vi "sv_Insert Swept THD Values.vi"(8 "scaled measurements in":T1 {"harmonic components [ratio]" format="%.2f"; "THD [ratio]" format="%.2f"; "FRF Measurements"."Im [response]" format="%.2f"; "FRF Measurements"."Re [response]" format="%.2f"; "FRF Measurements"."Im [stimulus]" format="%.2f"; "FRF Measurements"."Re [stimulus]" format="%.2f"; "RMS response" format="%.2f"; "RMS stimulus" format="%.2f"}, 10 "AI freq index":i32, 11 "measurements in":T2 {"scaled response magnitude" format="%.3f"; "Harm[]" format="%.2f"; "THD" format="%.2f"; "Im [response]" format="%.2f"; "Re [response]" format="%.2f"; "Im [stimulus]" format="%.2f"; "Re [stimulus]" format="%.2f"; "RMS response" format="%.2f"; "RMS stimulus" format="%.2f"}) -> (0 "dup new measurements":T1 {"harmonic components [ratio]" format="%.2f"; "THD [ratio]" format="%.2f"; "FRF Measurements"."Im [response]" format="%.2f"; "FRF Measurements"."Re [response]" format="%.2f"; "FRF Measurements"."Im [stimulus]" format="%.2f"; "FRF Measurements"."Re [stimulus]" format="%.2f"; "RMS response" format="%.2f"; "RMS stimulus" format="%.2f"}, 2 "dup AI freq index":i32, 3 "measurements out":T2 {"scaled response magnitude" format="%.3f"; "Harm[]" format="%.2f"; "THD" format="%.2f"; "Im [response]" format="%.2f"; "Re [response]" format="%.2f"; "Im [stimulus]" format="%.2f"; "Re [stimulus]" format="%.2f"; "RMS response" format="%.2f"; "RMS stimulus" format="%.2f"})   [LabVIEW 2017, in "SoundVib_SweptSine.lvlib"]
uses:
  <vilib>/addons/Sound and Vibration/svt_Swept Sine/SoundVib_SweptSine.lvlib
  <vilib>/addons/Sound and Vibration/svt_Swept Sine/subVIs/sv_Swept Sine Measurements.ctl
panel:
  out "error out":errorcluster
  in  "error in (no error)":errorcluster
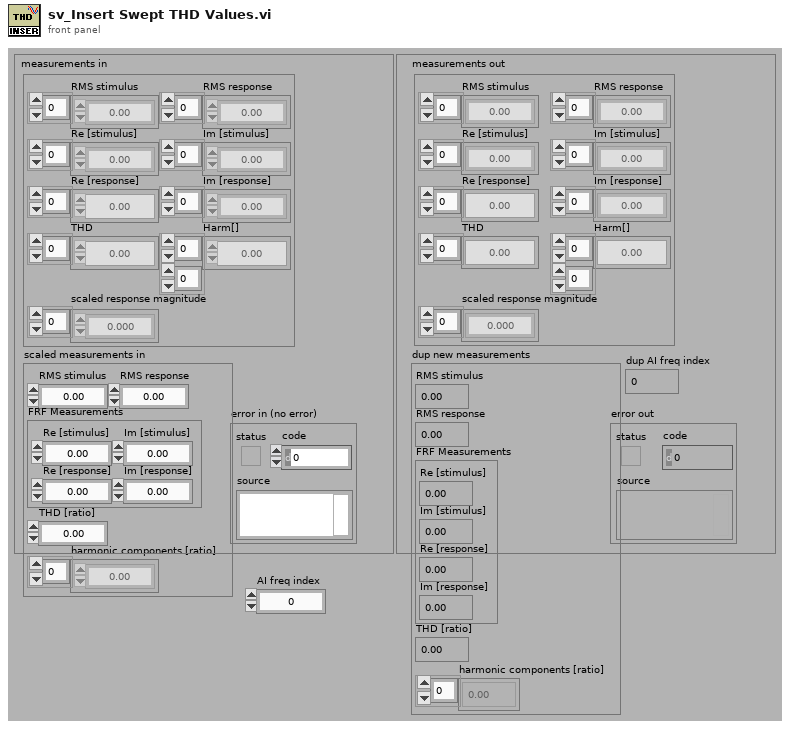
[diagram p1: front panel]
types:
  T1 = cluster{"RMS stimulus":dbl, "RMS response":dbl, "FRF Measurements":cluster{"Re [stimulus]":dbl, "Im [stimulus]":dbl, "Re [response]":dbl, "Im [response]":dbl}, "THD [ratio]":dbl, "harmonic components [ratio]":dbl[]}
  T2 = typedef "SoundVib_SweptSine.lvlib/sv_Swept Sine Measurements.ctl" = cluster{"RMS stimulus":dbl[], "RMS response":dbl[], "Re [stimulus]":dbl[], "Im [stimulus]":dbl[], "Re [response]":dbl[], "Im [response]":dbl[], "THD":dbl[], "Harm[]":dbl[][], "scaled response magnitude":dbl[]}
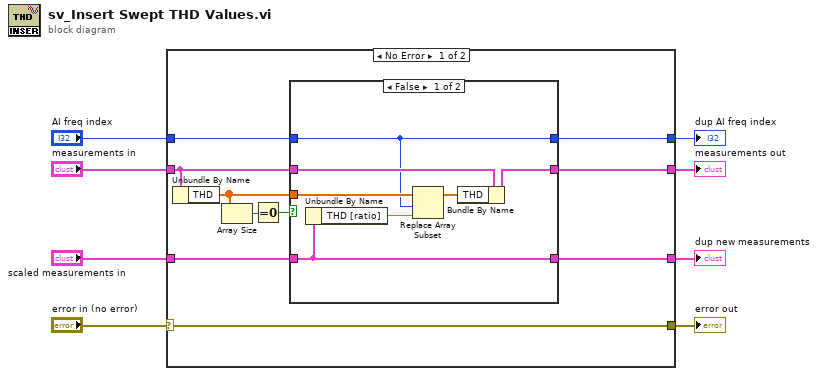
[diagram p0: block diagram]
diagram:
  n1 = case shown="No Error" "error in (no error)" {
    selector: "error in (no error)" -> [w13 w32]
    tunnel: "measurements in" -> [w16 w31]
    tunnel: [w14 w31] -> w7
    tunnel: [w13 w32] -> w5
    tunnel: "scaled measurements in" -> [w11 w30]
    tunnel: "AI freq index" -> [w12 w29]
    tunnel: [w10 w30] -> w3
    tunnel: [w9 w29] -> w1
    frame No Error {
      n2 = Unbundle By Name(w16) -> ("THD"=w18:dbl[])
      n3 = Array Size(array=w18) -> (size(s)=w17:i32)
      n4 = Equal To 0?(x=w17) -> (x = 0?=w15:bool)
      n5 = case shown="False" w15 {
        tunnel: w16 -> [w22 w28]
        tunnel: [w21 w28] -> w14
        tunnel: w18 -> [w24 _]
        tunnel: w12 -> [w19 w26]
        tunnel: w11 -> [w20 w27]
        tunnel: [w20 w27] -> w10
        tunnel: [w19 w26] -> w9
        frame False {
          n6 = Unbundle By Name(w20) -> ("THD [ratio]"=w25:dbl)
          n7 = Replace Array Subset(array=w24, new element=w25, index=w19) -> (w23:dbl[])
          n8 = Bundle By Name(cluster=w22, "THD"=w23) -> (w21:T2)
        }
        frame True {
        }
      }
    }
    frame Error {
    }
  }
  "error out" <- w5
  "measurements out" <- w7
  "dup new measurements" <- w3
  "dup AI freq index" <- w1
